vi "main.vi"() -> ()   [LabVIEW 2018]
panel:
  in  "Default True":bool=TRUE
  in  "Open SubVI":bool
  in  "Stop Program":bool
  in  "Select SubVI":enum16{"SubVI 1", "SubVI 2", "SubVI 3"}(ring)
  # "Adapted from\nhttps://www.youtube.com/watch?v=jl0wTeN954A"
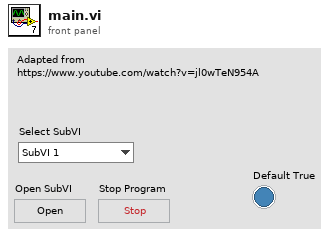
[diagram p1: front panel]
types:
  T1 = enum32{"Invalid", "Standard", "Closed", "Hidden", "Minimized", "Maximized"}
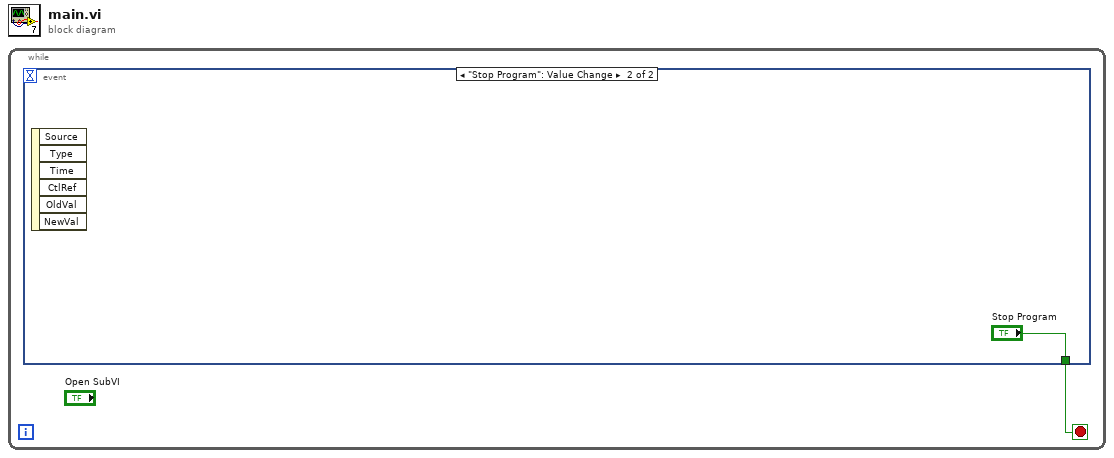
[diagram p0: block diagram]
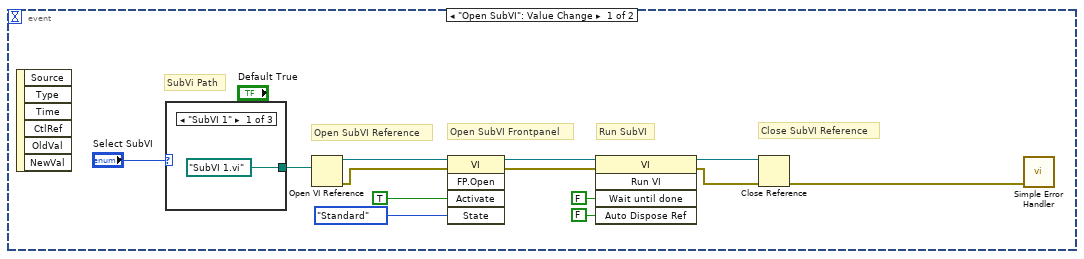
[diagram p2: hidden frame]
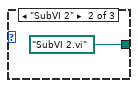
[diagram p3: hidden frame]
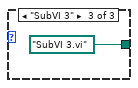
[diagram p4: hidden frame]
diagram:
  n1 = while {
    stop <- w1 stop-if-true
    n2 = event shown="[1] \"Stop Program\": Value Change" {
      selector: _ -> [_ _]
      dyn-events: _ -> [_ _]
      timeout: _ -> [_ _]
      tunnel: [_ "Stop Program"] -> w1
      event "Open SubVI": Value Change {
        # "Close SubVI Reference"
        # "Run SubVI"
        # "Open SubVI Frontpanel"
        # "Open SubVI Reference"
        # "SubVi Path"
        n3 = event-data() -> ()  [unwired: 1 in, 6 out]
        n4 = case shown="\"SubVI 1\"" "Select SubVI" {
          tunnel: [path "SubVI 1.vi" ("vi path") path "SubVI 2.vi" ("vi path") path "SubVI 3.vi" ("vi path")] -> w14
          frame "SubVI 1" {
          }
          frame "SubVI 2" {
          }
          frame "SubVI 3" {
          }
        }
        n5 = Open VI Reference(vi path=w14) -> (vi reference=w11:refnum<vi>, error out=w10:errorcluster)  [unwired: 5 in]
        n6 = invoke class="VI" method="FP.Open"(reference=w11, error in=w10, "Activate"=TRUE ("Activate?"), "State"=T1."Standard") -> (reference out=w13:refnum<vi>, error out=w12:errorcluster)  [unwired: 1 in, 3 out]
        n7 = invoke class="VI" method="Run VI"(reference=w13, error in=w12, "Wait until done"=FALSE ("Wait Until Done"), "Auto Dispose Ref"=FALSE ("Auto Dispose Reference")) -> (reference out=w9:refnum<vi>, error out=w8:errorcluster)  [unwired: 1 in, 3 out]
        n8 = Close Reference(reference=w9, error in (no error)=w8) -> (error out=w2:errorcluster)
        n9 = call <vilib>:"Simple Error Handler.vi"("error in (no error)"=w2) -> ()  [unwired: 4 in, 5 out]
      }
      event "Stop Program": Value Change {
        n10 = event-data() -> ()  [unwired: 1 in, 6 out]
      }
    }
  }
